vi "3-5-1.vi"() -> ()   [LabVIEW 2016]
uses:
  <vilib>/picture/picture.llb/imagedata.ctl
  <vilib>/Analysis/2dsp.llb/2D Convolution (DBL).vi
  <vilib>/picture/picture.llb/Draw 8-Bit Pixmap.vi
  <vilib>/Analysis/NI_AALPro.lvlib
panel:
  out "new picture 3":picture
  in  "output image":path
  out "new picture 2":picture
  out "new picture":picture
  out "image data":T1
  in  "input image":path
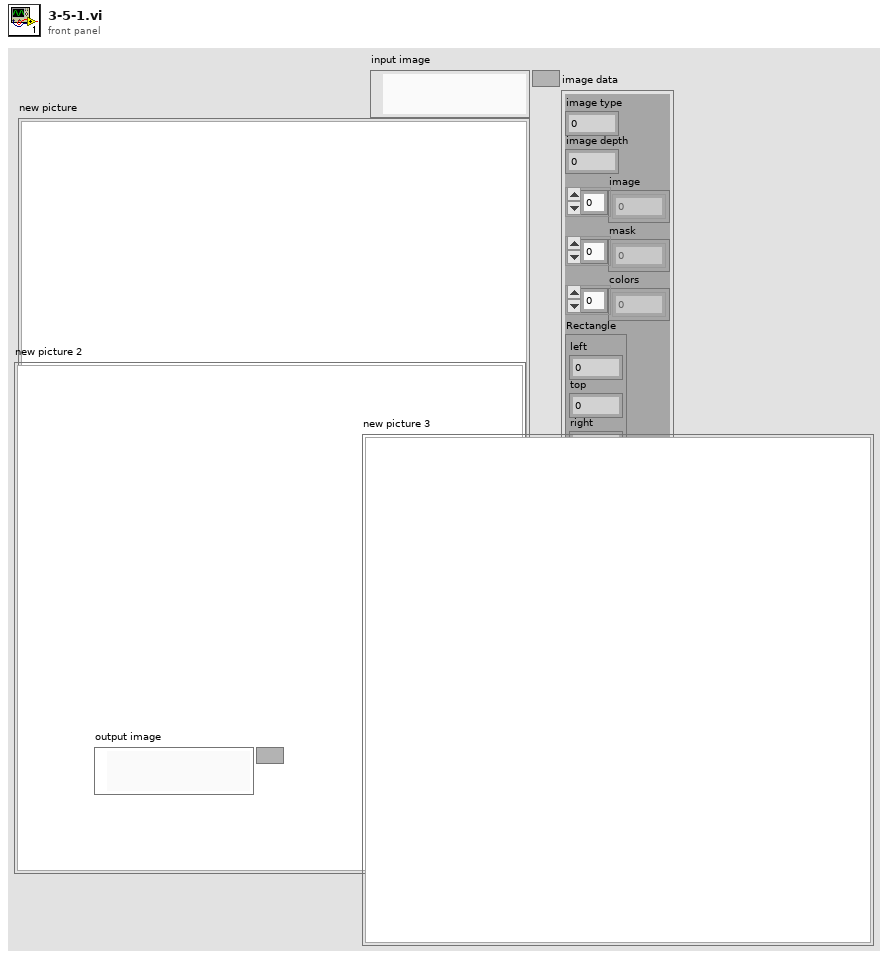
[diagram p1: front panel]
types:
  T1 = typedef "imagedata.ctl" = cluster{"image type":i32, "image depth":i32, "image":u8[], "mask":u8[], "colors":u32[], "Rectangle":cluster{"left":i16, "top":i16, "right":i16, "bottom":i16}}
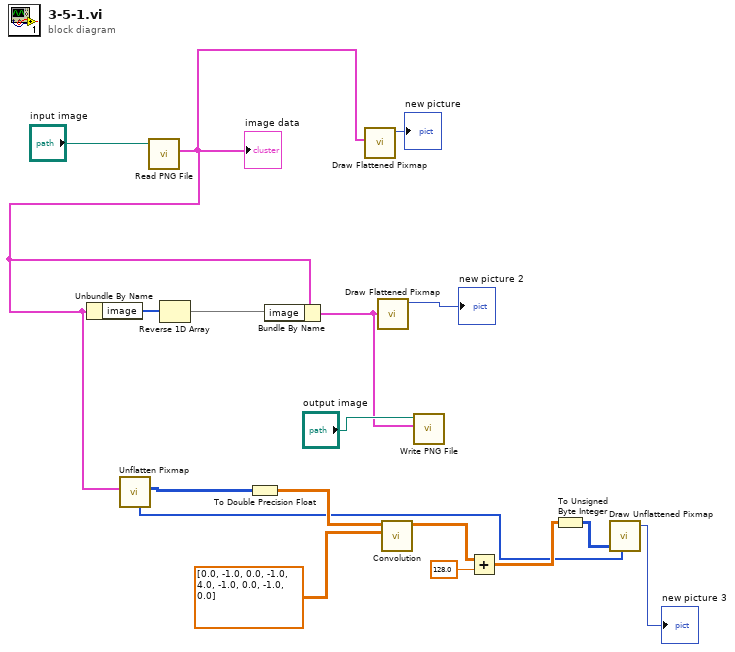
[diagram p0: block diagram]
diagram:
  n1 = call <vilib>:"Read PNG File.vi"("path to PNG file"="input image") -> ("image data"=w10:T1)  [unwired: 8 in, 2 out]
  "image data" <- w10
  n2 = Unbundle By Name(w10) -> ("image"=w15:u8[])
  n3 = call <vilib>:"Unflatten Pixmap.vi"("image data"=w10) -> ("8-bit pixmap"=w9:u8[][], "colors"=w1:u32[])  [unwired: 4 in, 5 out]
  n4 = Reverse 1D Array(array=w15) -> (reversed array=w14:u8[])
  n5 = To Double Precision Float(number=w9) -> (double precision float=w8:dbl[][])
  n6 = Bundle By Name(cluster=w10, "image"=w14) -> (w11:T1)
  n7 = call <vilib>:"Draw Flattened Pixmap.vi"("image data"=w10) -> ("new picture"=→"new picture":picture)  [unwired: 8 in]
  n8 = call <vilib>:"Draw Flattened Pixmap.vi"("image data"=w11) -> ("new picture"=→"new picture 2":picture)  [unwired: 8 in]
  n9 = call-poly <vilib>:"Convolution.vi"("Y"=dbl[][] [[0.0, -1.0, 0.0], [-1.0, 4.0, -1.0], [0.0, -1.0, 0.0]], "X"=w8) -> ("X * Y"=w5:dbl[][])  [unwired: 8 in, 1 out]
  n10 = call <vilib>:"Write PNG File.vi"("image data"=w11, "path to PNG file"="output image") -> ()  [unwired: 8 in, 2 out]
  n11 = Add(x=w5, y=128.0) -> (x+y=w4:dbl[][])
  n12 = To Unsigned Byte Integer(number=w4) -> (unsigned 8bit integer=w3:u8[][])
  n13 = call-poly <vilib>:"Draw Unflattened Pixmap.vi"("data"=w3, "color table"=w1) -> ("new picture"=→"new picture 3":picture)  [unwired: 7 in]
